vi "Integrator (DBL Array).vi"(2 "initialize":bool, 3 "dt":dbl=1e-09 min=1e-09 format="%.6f", 4 "initial conditions":dbl[](array[numeric]) format="%.2f", 5 "input points":dbl[](array[numeric]) format="%.2f") -> (1 "output points":dbl[](array[numeric]) format="%.2f")   [LabVIEW 2020, in "NI_AdvCtrl_continuous linear.lvlib"]
doc: "LabVIEW no longer supports this VI. You can obtain similar functionality by installing the LabVIEW Simulation Module.\n\nIntegrates a continuous input signal. The integration process is based on Euler method. dt must be positive."
uses:
  <vilib>/addons/control/advanced/NI_AdvCtrl_continuous linear.lvlib
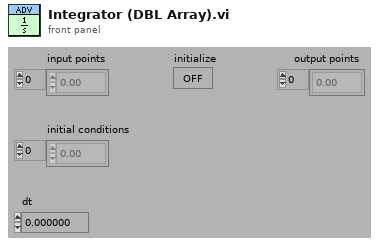
[diagram p1: front panel]
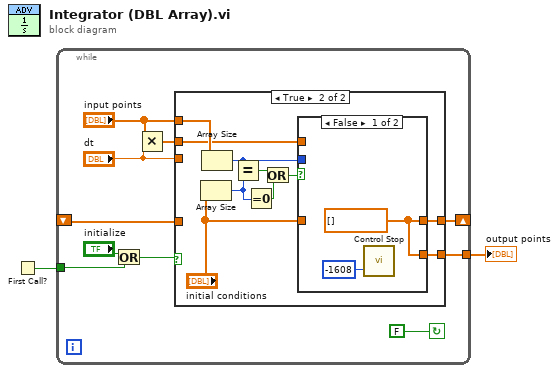
[diagram p0: block diagram]
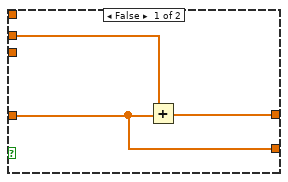
[diagram p2: hidden frame]
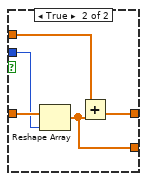
[diagram p3: hidden frame]
diagram:
  n1 = First Call?() -> (First Call?: T/F=w2:bool)
  n2 = while {
    tunnel: [w3] -> w1
    tunnel: w2 -> [w8]
    shift-left: _ -> [w11]
    shift-right: [w12] -> _
    stop <- FALSE continue-if-true
    n3 = Or(x="initialize", y=w8) -> (x .or. y?=w7:bool)
    n4 = Multiply(x="input points", y="dt") -> (x*y=w4:dbl[])
    n5 = case shown="True" w7 {
      tunnel: [w15 w24] -> w12
      tunnel: "input points" -> [_ w25]
      tunnel: w11 -> [w13 _]
      tunnel: "dt" -> [_ _]
      tunnel: w4 -> [w14 w22]
      tunnel: [w13 w16] -> w3
      frame False {
        n6 = Add(x=w14, y=w13) -> (x+y=w15:dbl[])
      }
      frame True {
        n7 = Array Size(array="initial conditions") -> (size(s)=w21:i32)
        n8 = Array Size(array=w25) -> (size(s)=w17:i32)
        n9 = Equal?(x=w17, y=w21) -> (x = y?=w19:bool)
        n10 = Equal To 0?(x=w21) -> (x = 0?=w18:bool)
        n11 = Or(x=w19, y=w18) -> (x .or. y?=w20:bool)
        n12 = case shown="False" w20 {
          tunnel: "initial conditions" -> [_ w32]
          tunnel: [w26 w30] -> w24
          tunnel: w22 -> [_ w31]
          tunnel: w17 -> [_ w29]
          tunnel: [w26 w28] -> w16
          frame False {
            w26 = dbl[] [] ("Initial Conditions")
            n13 = call <vilib>:"Control Stop.vi"("error"=-1608) -> ()  [unwired: 2 out]
          }
          frame True {
            n14 = Reshape Array(w32, w29) -> (w28:dbl[])
            n15 = Add(x=w31, y=w28) -> (x+y=w30:dbl[])
          }
        }
      }
    }
  }
  "output points" <- w1
